vi "GlobalData7.vi"(3 "1D Input Array":sgl[](array[numeric]), 4 "1D Time Array":sgl[](array[numeric]), 5 "Function select":string) -> (0 "2D Output Time Array":sgl[][](array[numeric]), 1 "1D Output Array":sgl[](array[numeric]), 2 "2D Output Data Array":sgl[][](array[numeric]))   [LabVIEW 2013]
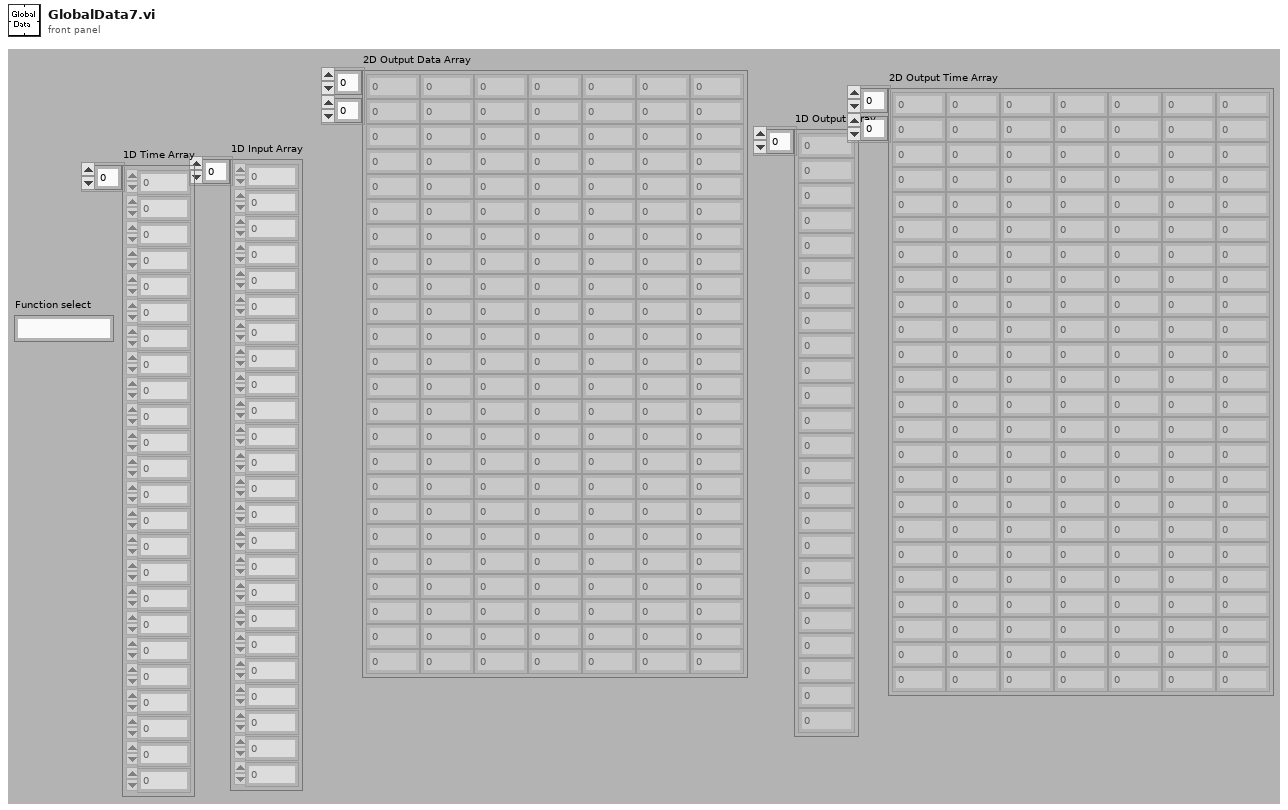
[diagram p1: front panel]
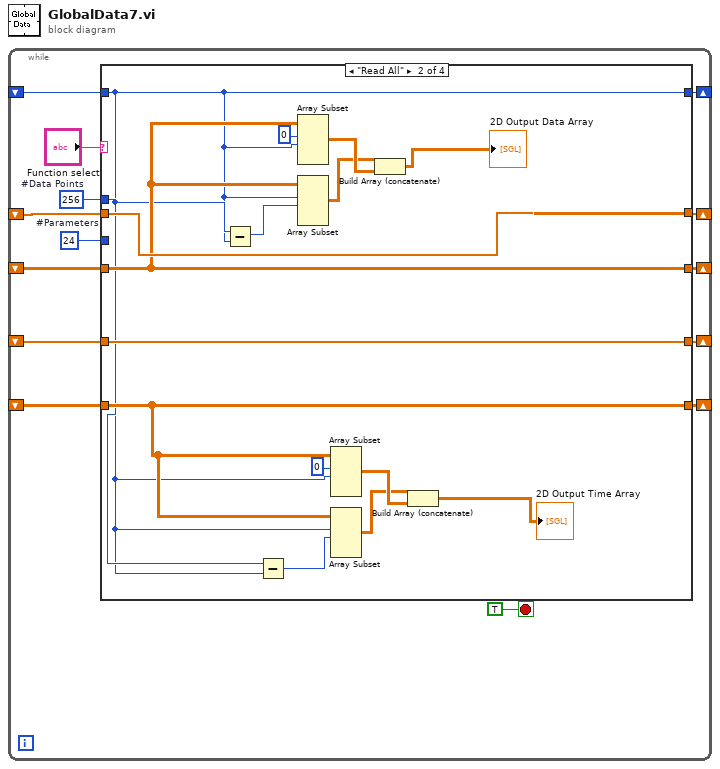
[diagram p0: block diagram]
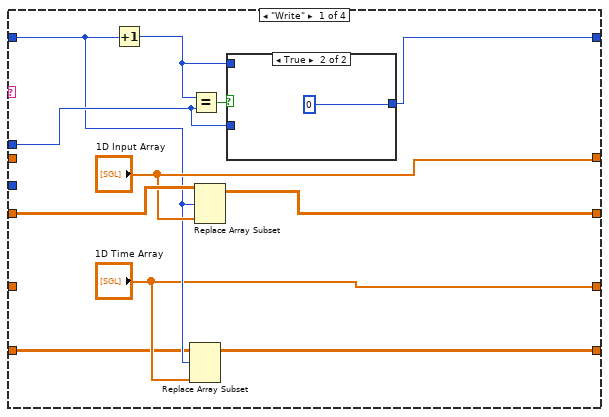
[diagram p2: hidden frame]
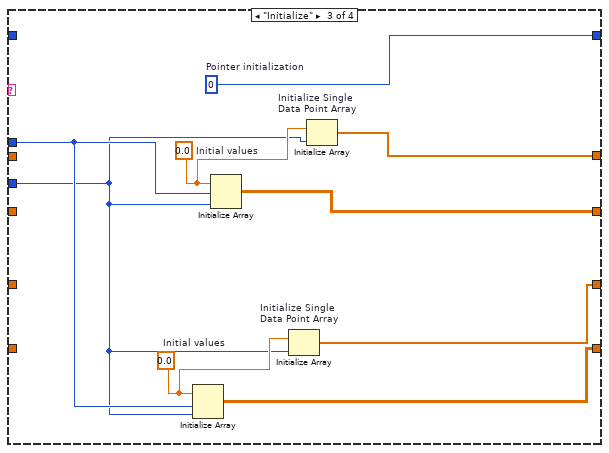
[diagram p4: hidden frame]
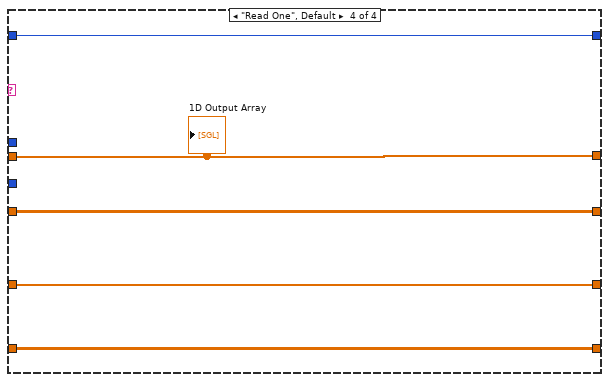
[diagram p5: hidden frame]
diagram:
  n1 = while {
    shift-right: [w12] -> _
    shift-left: _ -> [w10]
    shift-right: [w5] -> _
    shift-left: _ -> [w11]
    shift-right: [w7] -> _
    shift-left: _ -> [w6]
    shift-right: [w3] -> _
    shift-left: _ -> [w2]
    shift-right: [w4] -> _
    shift-left: _ -> [w1]
    stop <- TRUE stop-if-true
    w9 = 24  # #Parameters
    w8 = 256  # #Data Points
    n2 = case shown="\"Read All\"" "Function select" {
      tunnel: [w24 w29 w52 w56] -> w12
      tunnel: w11 -> [w25 w38 _ w55]
      tunnel: w10 -> [w18 w29 _ w56]
      tunnel: w9 -> [_ _ w44 _]
      tunnel: w8 -> [w21 w30 w47 _]
      tunnel: ["1D Input Array" w39 w49 w57] -> w7
      tunnel: w6 -> [_ w39 _ w57]
      tunnel: [w19 w38 w51 w55] -> w5
      tunnel: ["1D Time Array" w36 w46 w54] -> w4
      tunnel: w2 -> [w16 w31 _ w53]
      tunnel: [w15 w31 w45 w53] -> w3
      tunnel: w1 -> [_ w36 _ w54]
      frame "Write" {
        n3 = Increment(x=w18) -> (x+1=w22:u32)
        n4 = Replace Array Subset(array=w16, new element="1D Time Array", index (row)=w18) -> (w15:sgl[][])  [unwired: 1 in]
        n5 = Equal?(x=w22, y=w21) -> (x = y?=w23:bool)
        n6 = Replace Array Subset(array=w25, new element="1D Input Array", index (row)=w18) -> (w19:sgl[][])  [unwired: 1 in]
        n7 = case shown="True" w23 {
          tunnel: [w26 0] -> w24
          tunnel: w22 -> [w26 _]
          tunnel: w21 -> [_ _]
          frame False {
          }
          frame True {
          }
        }
      }
      frame "Read All" {
        n8 = Subtract(x=w30, y=w29) -> (x-y=w40:u32)
        n9 = Subtract(x=w30, y=w29) -> (x-y=w32:u32)
        n10 = Array Subset(array=w38, index (row)=0, length (row)=w29) -> (w43:sgl[][])  [unwired: 2 in]
        n11 = Array Subset(array=w38, index (row)=w29, length (row)=w40) -> (w42:sgl[][])  [unwired: 2 in]
        n12 = Array Subset(array=w31, index (row)=0, length (row)=w29) -> (w35:sgl[][])  [unwired: 2 in]
        n13 = Array Subset(array=w31, index (row)=w29, length (row)=w32) -> (w34:sgl[][])  [unwired: 2 in]
        n14 = Build Array (concatenate)(w42, w43) -> (→"2D Output Data Array":sgl[][])
        n15 = Build Array (concatenate)(w34, w35) -> (→"2D Output Time Array":sgl[][])
      }
      frame "Initialize" {
        w48 = sgl 0.0  # Initial values
        w52 = u32 0  # Pointer initialization
        w50 = sgl 0.0  # Initial values
        n16 = Initialize Array(w48, w47, w44) -> (w45:sgl[][])
        n17 = Initialize Array(w50, w47, w44) -> (w51:sgl[][])
        n18 = Initialize Array "Initialize Single\nData Point Array"(w48, w44) -> (w46:sgl[])
        n19 = Initialize Array "Initialize Single\nData Point Array"(w50, w44) -> (w49:sgl[])
      }
      frame "Read One", Default {
        "1D Output Array" <- w57
      }
    }
  }
